vi "Read Simple Command Status.vi"(11 "Device Activation Status Msg in":refnum<class "Simple Command Status Msg.lvclass">) -> (1 "Status":T1, 2 "error":string, 3 "Device Activation Status Msg out":refnum<class "Simple Command Status Msg.lvclass">)   [LabVIEW 2015, in "SCADA Core.lvlib" / "Simple Command Status Msg.lvclass"]
uses:
  Simple Command Status Msg.lvclass
  Simple Command Status.ctl
  Simple Command Status Msg.lvclass/Simple Command Status Msg.ctl
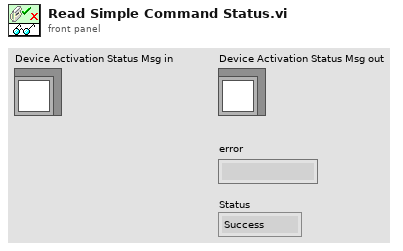
[diagram p1: front panel]
types:
  T1 = typedef "SCADA Core.lvlib/Simple Command Status Msg.lvclass/Simple Command Status.ctl" = enum16{"Success", "Failure"}
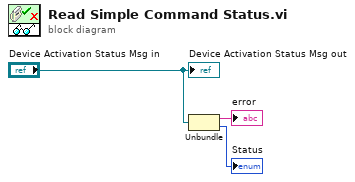
[diagram p0: block diagram]
diagram:
  n1 = Unbundle("Device Activation Status Msg in") -> (→"error":string, →"Status":T1)
  "Device Activation Status Msg out" <- "Device Activation Status Msg in"
